vi "fgv_rc-config.vi"(7 "cmd":T2, 8 "error in (no error)":errorcluster, 11 "Testconfig":T1={"Test Mode"=enum."6.3.2 저온 작동/방치 시험", "ON time[ms]"=200.0, "OFF time[ms]"=500.0, "1. 작동시간[분]"=10000.0, "2. 미작동시간[분]"=10000.0, "3. 작동시간[분]"=10000.0, "level[V]"=12.0, "duty"=20.0, "Freq"=1.0, "Voltage+[V]"=20.0, "Voltage-[V]"=-20.0, "Current+[A]"=5.0, "Current-[A]"=-5.0, "출력전압[V]"=200.0, "출력전류[A]"=10.0, "OVP Level"=0.0, "OCP Level"=0.0, "Time Div"=2, "Record Len"=5, "방전 기준[V]"=0.0, "Repeate (Each Ch)"=3, "Cycle[N]"=1, "ON/OFF 회 수[N]"=10000.0, "TrigPos[%]"=0.0, "시험시간[분]"=1.0} {"시험시간[분]" min=1.0; "ON/OFF 회 수[N]" min=1.0; "3. 작동시간[분]" min=1.0; "2. 미작동시간[분]" min=1.0; "1. 작동시간[분]" min=1.0; "Time Div" items=["10m", "20ms", "50ms", "100ms", "200ms", "500ms", "1s", "2s", "5s", "10s", "20s", "30s", "1min", "2min", "5min"]; "OFF time[ms]" min=10000.0 max=1000000.0; "Current-[A]" min=-20.0 max=20.0 step=0.001; "Voltage-[V]" min=-115.0 max=115.0 step=0.01; "Current+[A]" min=0.0 max=60.0 step=0.01; "Voltage+[V]" min=0.0 max=120.0 step=0.1; "OCP Level" format="%#_13g"; "OVP Level" format="%#_13g"; "Record Len" items=["10k", "25k", "50k", "100k", "250k", "500k", "1M", "2.5M", "5M", "10M", "25M", "50M", "100M", "250M", "500M", "1G", "2G", "4G", "5G", "10G", "20G", "50G"]; "ON time[ms]" min=50.0 max=2000000.0}) -> (0 "error out":errorcluster, 3 "Testconfig out":T1={"Test Mode"=enum."6.3.2 저온 작동/방치 시험", "ON time[ms]"=200.0, "OFF time[ms]"=500.0, "1. 작동시간[분]"=10000.0, "2. 미작동시간[분]"=10000.0, "3. 작동시간[분]"=10000.0, "level[V]"=12.0, "duty"=20.0, "Freq"=1.0, "Voltage+[V]"=20.0, "Voltage-[V]"=-20.0, "Current+[A]"=5.0, "Current-[A]"=-5.0, "출력전압[V]"=200.0, "출력전류[A]"=10.0, "OVP Level"=0.0, "OCP Level"=0.0, "Time Div"=2, "Record Len"=5, "방전 기준[V]"=0.0, "Repeate (Each Ch)"=3, "Cycle[N]"=1, "ON/OFF 회 수[N]"=10000.0, "TrigPos[%]"=0.0, "시험시간[분]"=1.0} {"시험시간[분]" min=1.0; "ON/OFF 회 수[N]" min=1.0; "3. 작동시간[분]" min=1.0; "2. 미작동시간[분]" min=1.0; "1. 작동시간[분]" min=1.0; "Time Div" items=["10m", "20ms", "50ms", "100ms", "200ms", "500ms", "1s", "2s", "5s", "10s", "20s", "30s", "1min", "2min", "5min"]; "OFF time[ms]" min=10000.0 max=1000000.0; "Current-[A]" min=-20.0 max=20.0 step=0.001; "Voltage-[V]" min=-115.0 max=115.0 step=0.01; "Current+[A]" min=0.0 max=60.0 step=0.01; "Voltage+[V]" min=0.0 max=120.0 step=0.1; "OCP Level" format="%#_13g"; "OVP Level" format="%#_13g"; "Record Len" items=["10k", "25k", "50k", "100k", "250k", "500k", "1M", "2.5M", "5M", "10M", "25M", "50M", "100M", "250M", "500M", "1G", "2G", "4G", "5G", "10G", "20G", "50G"]; "ON time[ms]" min=50.0 max=2000000.0})   [LabVIEW 2019]
uses:
  _ctrl/rw.ctl
  cap_config.ctl
panel:
  # "제어단 전압"
  # "출력단 전원"
  # "DL950"
  # "Discharge"
  # "Test Cycle"
  # "작동 설정"
  # "제어단 전압"
  # "출력단 전원"
  # "DL950"
  # "Discharge"
  # "Test Cycle"
  # "작동 설정"
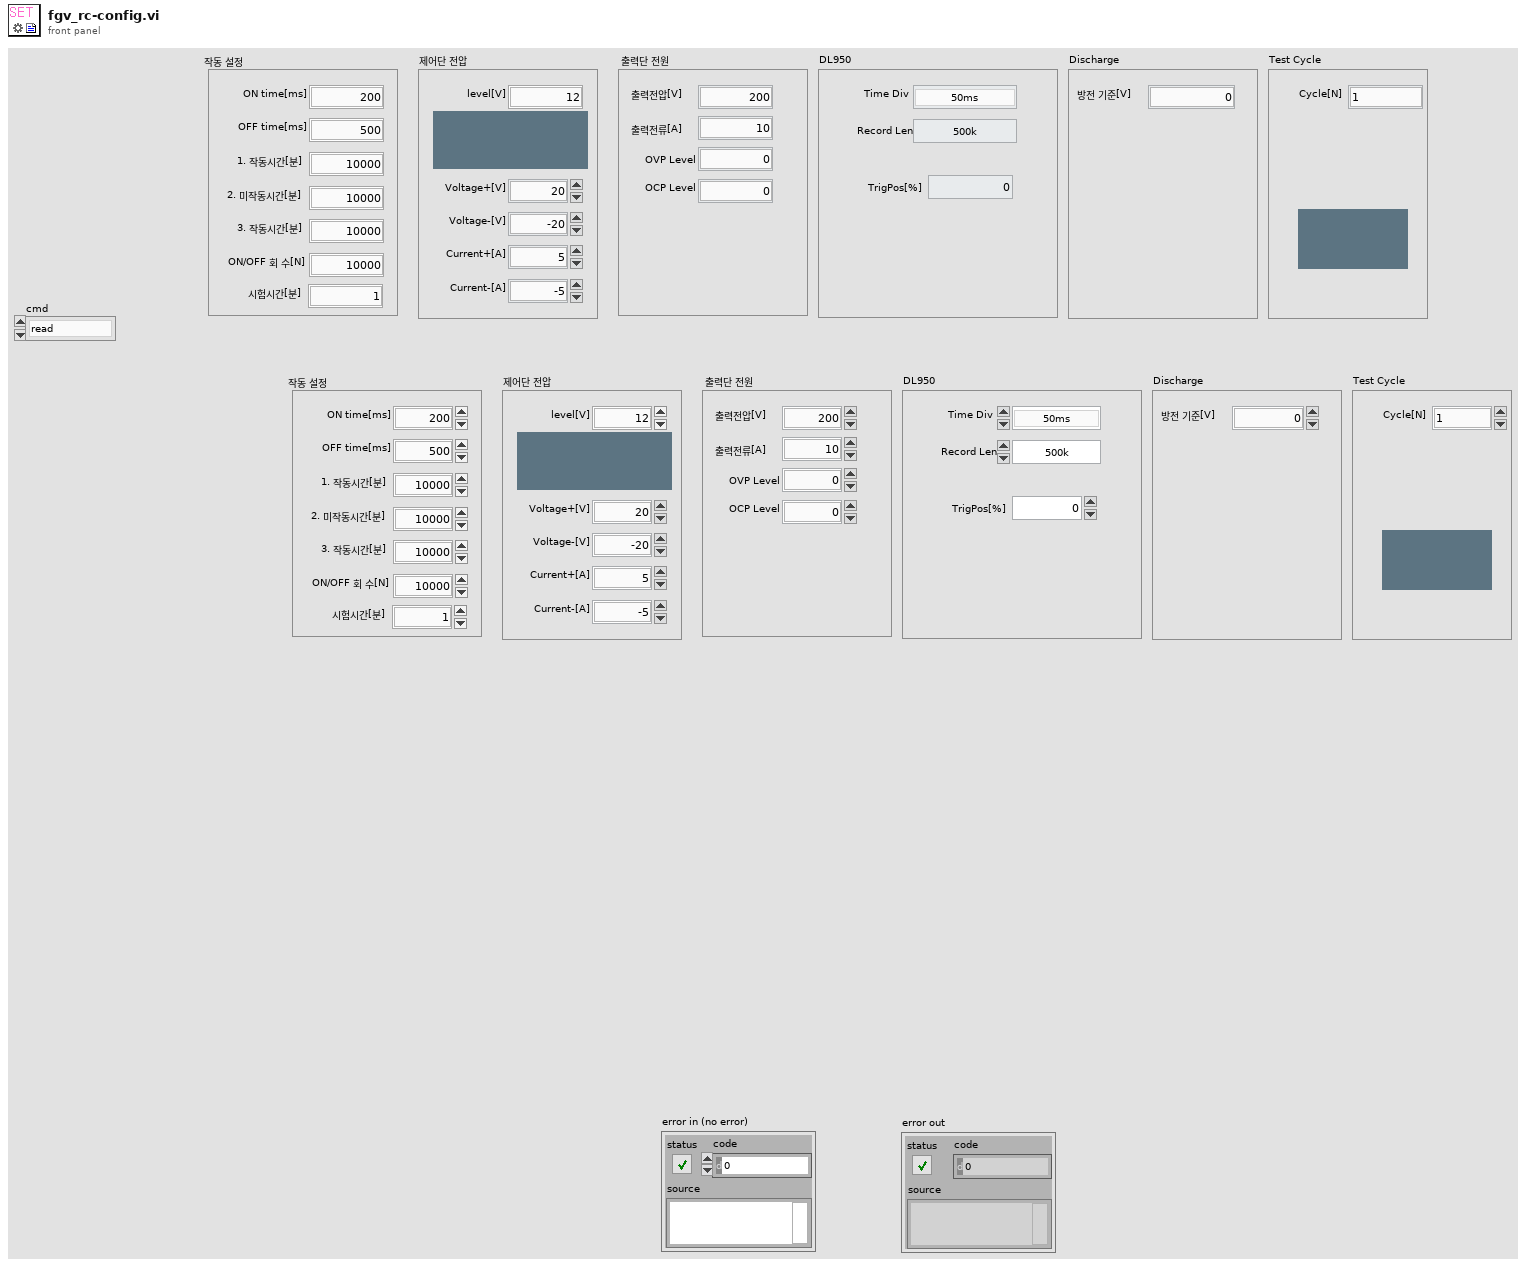
[diagram p1: front panel]
types:
  T1 = typedef "cap_config.ctl" = cluster{"Test Mode":enum32{"6.3.2 저온 작동/방치 시험", "6.3.3 고온 작동/방치 시험", "6.3.4 온도 싸이클 시험", "6.3.6 온습도 싸이클 시험", "6.3.8 결로 시험", "6.3.9 빙결 시험", "ON/OFF 동작시험"}, "ON time[ms]":dbl, "OFF time[ms]":dbl, "1. 작동시간[분]":dbl, "2. 미작동시간[분]":dbl, "3. 작동시간[분]":dbl, "level[V]":dbl, "duty":dbl, "Freq":dbl, "Voltage+[V]":dbl, "Voltage-[V]":dbl, "Current+[A]":dbl, "Current-[A]":dbl, "출력전압[V]":dbl, "출력전류[A]":dbl, "OVP Level":dbl, "OCP Level":dbl, "Time Div":u16, "Record Len":i32, "방전 기준[V]":dbl, "Repeate (Each Ch)":u32, "Cycle[N]":u32, "ON/OFF 회 수[N]":dbl, "TrigPos[%]":dbl, "시험시간[분]":dbl}
  T2 = typedef "rw.ctl" = enum16{"read", "write"}
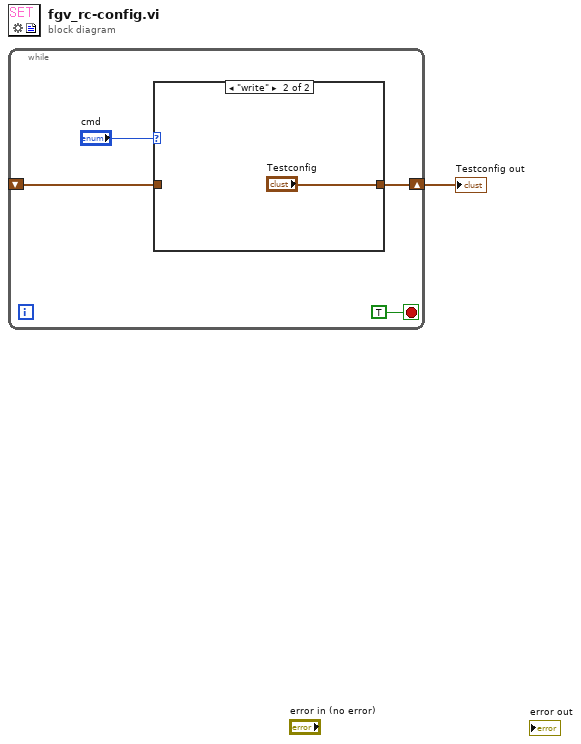
[diagram p0: block diagram]
diagram:
  n1 = while {
    shift-right: [w3] -> w1
    shift-left: _ -> [w2]
    stop <- TRUE stop-if-true
    n2 = case shown="\"write\"" "cmd" {
      tunnel: [w6 "Testconfig"] -> w3
      tunnel: w2 -> [w6 _]
      frame "read", Default {
      }
      frame "write" {
      }
    }
  }
  "Testconfig out" <- w1
